vi "Grid_ETA (SubVI).vi"(9 "points taken":i32, 10 "seconds since 1Jan1904":timestamp, 11 "points todo":i32) -> (1 "Numeric 4":dbl, 2 "Time Stamp":timestamp, 3 "Numeric 3":dbl)   [LabVIEW 2021]
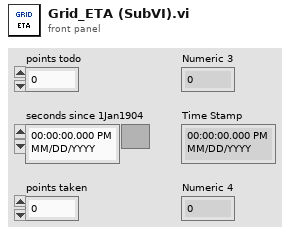
[diagram p1: front panel]
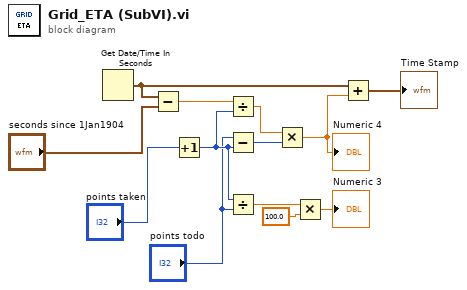
[diagram p0: block diagram]
diagram:
  n1 = Get Date/Time In Seconds() -> (seconds since 1Jan1904=w11:timestamp)
  n2 = Subtract(x=w11, y="seconds since 1Jan1904") -> (x-y=w12:dbl)
  n3 = Increment(x="points taken") -> (x+1=w13:i32)
  n4 = Divide(x=w12, y=w13) -> (x/y=w4:dbl)
  n5 = Subtract(x="points todo", y=w13) -> (x-y=w3:i32)
  n6 = Divide(x=w13, y="points todo") -> (x/y=w7:dbl)
  n7 = Multiply(x=w4, y=w3) -> (x*y=w1:dbl)
  "Numeric 4" <- w1
  n8 = Multiply(x=w7, y=100.0) -> (x*y=→"Numeric 3":dbl)
  n9 = Add(x=w11, y=w1) -> (x+y=→"Time Stamp":timestamp)
